vi "pad.vi"(8 "data length":i32, 11 "Last Block":u8[](array[numeric]) format="%02x") -> (2 "blocks":i32, 3 "Padding":u8[](array[numeric]) format="%02x")   [LabVIEW 2013, in "SHA-1.lvlib" / "SHA-1.lvclass"]
doc: "This VI creates a new string that represents the padding for the message string. The sum of the lengths of the message string and the padding string (in bytes) must be a multiple of 64."
uses:
  SHA-1.lvclass
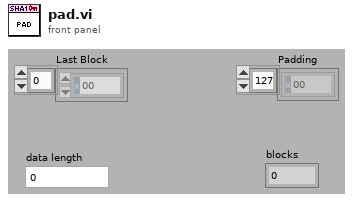
[diagram p1: front panel]
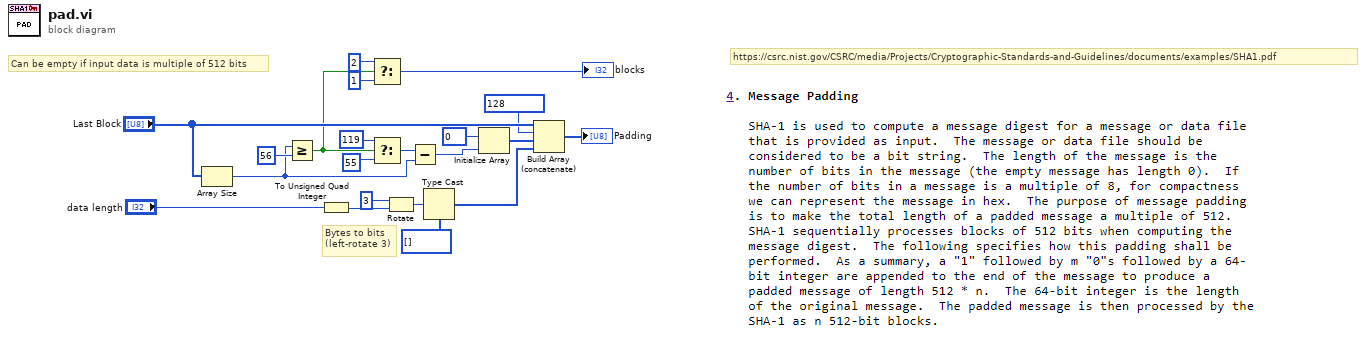
[diagram p0: block diagram]
diagram:
  # "https://csrc.nist.gov/CSRC/media/Projects/Cryptographic-Standards-and-Guidelines/documents/examples/SHA1.pdf"
  # "Bytes to bits\n(left-rotate 3)"
  # "Can be empty if input data is multiple of 512 bits"
  n1 = Array Size(array="Last Block") -> (size(s)=w11:i32)
  n2 = Greater Or Equal?(x=w11, y=56) -> (x >= y?=w6:bool)
  n3 = To Unsigned Quad Integer(1:"data length") -> (0:w21:u64)
  n4 = Select(t=2 ("blocks"), s=w6, f=1 ("blocks")) -> (s? t:f=→"blocks":i32)
  n5 = Select(t=119 ("dimension size"), s=w6, f=55 ("dimension size")) -> (s? t:f=w10:i32)
  n6 = Rotate(1:w21, 2:i16 3 ("y")) -> (0:w18:u64)
  n7 = Subtract(x=w10, y=w11) -> (x-y=w9:i32)
  n8 = Type Cast(type=u8[] [] ("Last Block"), x=w18) -> (*(type *) &x=w2:u8[])
  n9 = Initialize Array(u8 0, w9) -> (w7:u8[])
  n10 = Build Array (concatenate)("Last Block", u8 128, w7, w2) -> (→"Padding":u8[])
